vi "Find DAQ Devices.vi"(8 "Error In":errorcluster) -> (0 "Error Out":errorcluster, 2 "Stop?":bool, 3 "DAQmx Device Name":tag)   [LabVIEW 2017]
doc: "This VI returns information on all DAQ devices connected to the development computer. \n\nIf you do not wire any of the search inputs it will not return an element. It will, however, return the list of connected devices and serial numbers and a table of all the devices connected."
uses:
  <resource>/objmgr/daqmx.rc
panel:
  in  "OK Button":bool=TRUE
  in  "ConnectedDevices":u16(ring)
  out "All Device IDs":tag[](array[tag])
  # "Please select the correct connected device from the list:"
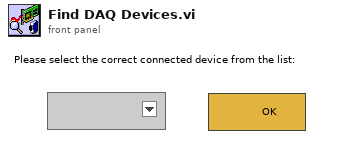
[diagram p1: front panel]
types:
  T1 = enum32{"Invalid", "Standard", "Closed", "Hidden", "Minimized", "Maximized"}
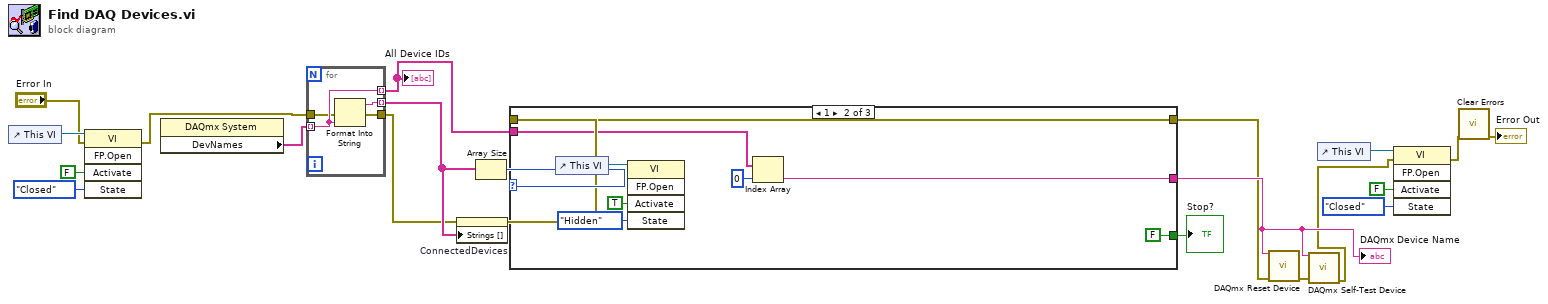
[diagram p0: block diagram]
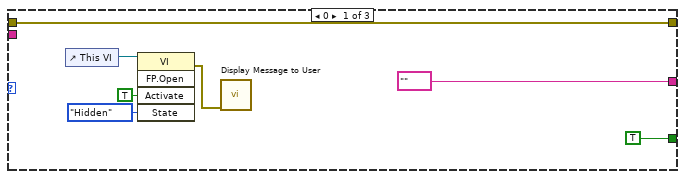
[diagram p2: hidden frame]
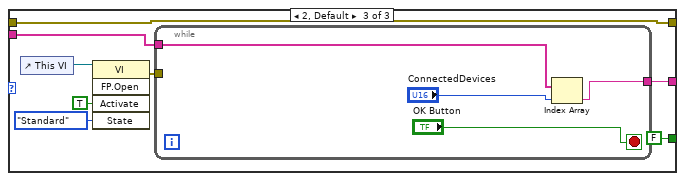
[diagram p3: hidden frame]
diagram:
  n1 = control-ref of="This VI"() -> (w11:refnum<vi>)
  n2 = invoke class="VI" method="FP.Open"(reference=w11, error in="Error In", "Activate"=FALSE ("Activate?"), "State"=T1."Closed") -> (error out=w9:errorcluster)  [unwired: 1 in, 4 out]
  n3 = property class="DAQmx System"() -> ("DevNames"=w21:tag[])  [unwired: 2 in, 2 out]
  n4 = for {
    tunnel: w21 -> [w24] mode=indexing
    tunnel: [w25] -> w20 mode=indexing
    tunnel: [w24] -> w18 mode=indexing
    tunnel: w9 -> [w23]
    tunnel: [w22] -> w8
    n5 = Format Into String(error in=w23, w24) -> (resulting string=w25:string, error out=w22:errorcluster)  [unwired: 2 in]
  }
  "All Device IDs" <- w18
  n6 = property on="ConnectedDevices" class="Ring (strict)"(error in=w8, "Strings []"=w20) -> (error out=w7:errorcluster)  [unwired: 1 in, 1 out]
  n7 = Array Size(array=w20) -> (size(s)=w19:i32)
  n8 = case shown="1" w19 {
    tunnel: w18 -> [_ w40 w47]
    tunnel: [tag "" w38 w46] -> w3
    tunnel: w7 -> [w31 w37 w48]
    tunnel: [w31 w37 w48] -> w2
    tunnel: [TRUE FALSE FALSE] -> w5
    frame 0 {
      n9 = control-ref of="This VI"() -> (w29:refnum<vi>)
      n10 = invoke class="VI" method="FP.Open"(reference=w29, "Activate"=TRUE ("Activate?"), "State"=T1."Hidden") -> (error out=w26:errorcluster)  [unwired: 2 in, 4 out]
      n11 = call "Display Message to User"("error in (no error)"=w26) -> ()  [unwired: 9 in, 2 out]
    }
    frame 1 {
      n12 = control-ref of="This VI"() -> (w35:refnum<vi>)
      n13 = invoke class="VI" method="FP.Open"(reference=w35, "Activate"=TRUE ("Activate?"), "State"=T1."Hidden") -> ()  [unwired: 2 in, 5 out]
      n14 = Index Array(array=w40, index=0) -> (element=w38:tag)
    }
    frame 2, Default {
      n15 = control-ref of="This VI"() -> (w43:refnum<vi>)
      n16 = invoke class="VI" method="FP.Open"(reference=w43, "Activate"=TRUE ("Activate?"), "State"=T1."Standard") -> (error out=w42:errorcluster)  [unwired: 2 in, 4 out]
      n17 = while {
        tunnel: w47 -> [w51]
        tunnel: [w50] -> w46
        tunnel: w42 -> [_]
        stop <- "OK Button" stop-if-true
        n18 = Index Array(array=w51, index="ConnectedDevices") -> (element=w50:tag)
      }
    }
  }
  "DAQmx Device Name" <- w3
  "Stop?" <- w5
  n19 = call <vilib>:"DAQmx Reset Device.vi"("device in"=w3, "error in"=w2) -> ("error out"=w4:errorcluster)  [unwired: 13 in]
  n20 = call <vilib>:"DAQmx Self-Test Device.vi"("device in"=w3, "error in"=w4) -> ("error out"=w1:errorcluster)  [unwired: 13 in]
  n21 = control-ref of="This VI"() -> (w15:refnum<vi>)
  n22 = invoke class="VI" method="FP.Open"(reference=w15, error in=w1, "Activate"=FALSE ("Activate?"), "State"=T1."Closed") -> (error out=w14:errorcluster)  [unwired: 1 in, 4 out]
  n23 = call <vilib>:"Clear Errors.vi"("error in (no error)"=w14) -> ("error out"=→"Error Out":errorcluster)  [unwired: 5 in, 1 out]
